vi "S2C_VLFT10_Proc_WaitForReboot.vi"(7 "Timeout":dbl, 8 "Error In":errorcluster, 11 "State":string) -> (0 "Error Out":errorcluster, 3 "Result":string)   [LabVIEW 2015]
uses:
  Fornax/VIs/PolyDriver/Typedefs/ExternalCommClient.ctl
  Fornax/VIs/PolyDriver/Typedefs/SystemState.ctl
  Fornax/VIs/S2C_FORNAX_Proc_Globals.vi
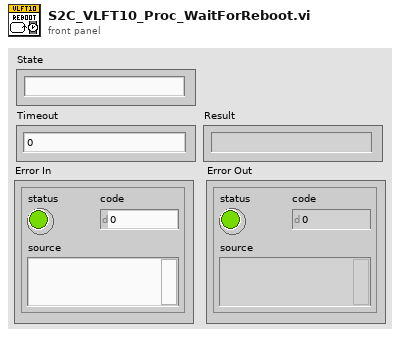
[diagram p1: front panel]
types:
  T1 = typedef "ExternalCommClient.ctl" = i16
  T2 = cluster{"ClientType":T1, "PostDelay (ms)":i32, "ClearFornaxMsgs":bool}
  T3 = cluster{"Partition":string, "Message":string, "M_ClientType":T1, "M_ClientId":string, "M_ResponseVersion":string, "M_ControllerBoardId":string, "M_ResponseValue":string, "M_ClientAlias":string, "M_ResponseOptions":string, "M_ClientIpAddress":string, "M_Crc32":i32}
  T4 = cluster{"Partition":string, "Message":string, "M_ClientType":T1, "M_ClientId":string, "M_ResponseVersion":string, "M_ControllerBoardId":string, "M_ResponseValue":string, "M_ClientAlias":string, "M_ResponseOptions":string, "M_ClientIpAddress":string}
  T5 = typedef "SystemState.ctl" = i16
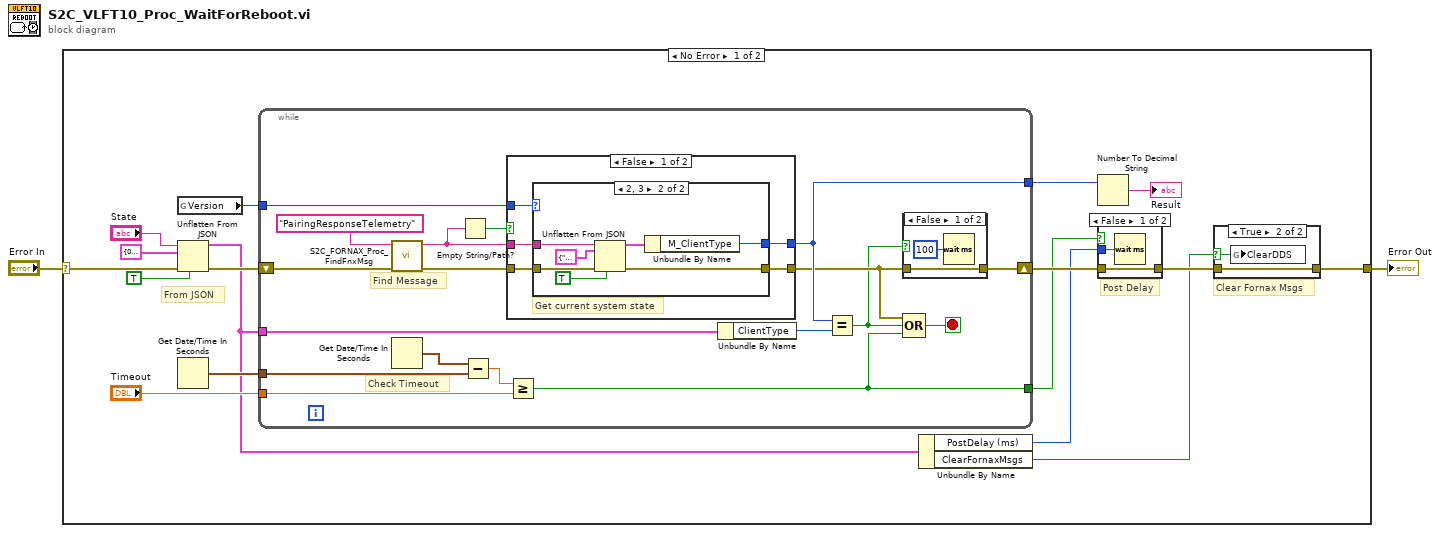
[diagram p0: block diagram]
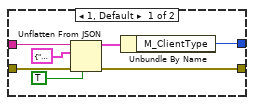
[diagram p5: hidden frame]
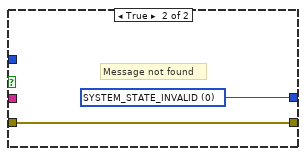
[diagram p6: hidden frame]
diagram:
  n1 = case shown="No Error" "Error In" {
    selector: "Error In" -> [w16 w68]
    tunnel: [w5 w68] -> w1
    frame No Error {
      # "Clear Fornax Msgs"
      # "Post Delay"
      # "From JSON"
      n2 = global read "S2C_FORNAX_Proc_Globals.vi" "Version"() -> (w19:i32)
      n3 = Unflatten From JSON(JSON string="State", type and defaults=T2 {"ClientType"=0, "PostDelay (ms)"=0, "ClearFornaxMsgs"=FALSE}, default null elements? (F)=TRUE, error in (no error)=w16) -> (value=w10:T2, error out=w15:errorcluster)  [unwired: 3 in]
      n4 = Get Date/Time In Seconds() -> (seconds since 1Jan1904=w14:timestamp)
      n5 = while {
        tunnel: w19 -> [w42]
        tunnel: w10 -> [w40]
        shift-right: [w29] -> w9
        shift-left: w15 -> [w41]
        tunnel: w14 -> [w36]
        tunnel: "Timeout" -> [w35]
        tunnel: [w31] -> w12
        tunnel: [w27] -> w8
        stop <- w32 stop-if-true
        # "Check Timeout"
        # "Find Message"
        n6 = call "S2C_FORNAX_Proc_FindFnxMsg.vi"("Error In"=w41, "MsgName"="PairingResponseTelemetry") -> ("Error Out"=w43:errorcluster, "Message"=w38:string)  [unwired: 8 in]
        n7 = Get Date/Time In Seconds() -> (seconds since 1Jan1904=w37:timestamp)
        n8 = Empty String/Path?(string/path=w38) -> (empty?=w39:bool)
        n9 = Subtract(x=w37, y=w36) -> (x-y=w34:dbl)
        n10 = case shown="False" w39 {
          tunnel: w43 -> [w51 w67]
          tunnel: w42 -> [w50 _]
          tunnel: [w49 w67] -> w30
          tunnel: [w48 w66] -> w31
          tunnel: w38 -> [w47 _]
          frame False {
            # "Get current system state"
            n11 = case shown="2, 3" w50 {
              tunnel: w51 -> [w57 w64]
              tunnel: [w55 w62] -> w49
              tunnel: [w54 w61] -> w48
              tunnel: w47 -> [w53 w60]
              frame 1, Default {
                n12 = Unflatten From JSON(JSON string=w53, type and defaults=T3 {"Partition"="", "Message"="", "M_ClientType"=0, "M_ClientId"="", "M_ResponseVersion"="", "M_ControllerBoardId"="", "M_ResponseValue"="", "M_ClientAlias"="", "M_ResponseOptions"="", "M_ClientIpAddress"="", "M_Crc32"=0}, default null elements? (F)=TRUE, error in (no error)=w57) -> (value=w56:T3, error out=w55:errorcluster)  [unwired: 3 in]
                n13 = Unbundle By Name(w56) -> ("M_ClientType"=w54:T1)
              }
              frame 2, 3 {
                n14 = Unflatten From JSON(JSON string=w60, type and defaults=T4 {"Partition"="", "Message"="", "M_ClientType"=0, "M_ClientId"="", "M_ResponseVersion"="", "M_ControllerBoardId"="", "M_ResponseValue"="", "M_ClientAlias"="", "M_ResponseOptions"="", "M_ClientIpAddress"=""}, default null elements? (F)=TRUE, error in (no error)=w64) -> (value=w63:T4, error out=w62:errorcluster)  [unwired: 3 in]
                n15 = Unbundle By Name(w63) -> ("M_ClientType"=w61:T1)
              }
            }
          }
          frame True {
            w66 = T5 0 items=["SYSTEM_STATE_INVALID", "SYSTEM_STATE_INIT", "SYSTEM_STATE_POST", "SYSTEM_STATE_CLINICAL", "SYSTEM_STATE_SERVICE", "SYSTEM_STATE_SW_UPDATE", "SYSTEM_STATE_SHUTDOWN", "SYSTEM_STATE_CALIBRATION", "SYSTEM_STATE_CONFIGURATION", "SYSTEM_STATE_CLINICAL_CONFIGURATION"] ("M_SystemState")
            # "Message not found"
          }
        }
        n16 = Greater Or Equal?(x=w34, y=w35) -> (x >= y?=w27:bool)
        n17 = Unbundle By Name(w40) -> ("ClientType"=w33:T1)
        n18 = Equal?(x=w31, y=w33) -> (x = y?=w28:bool)
        n19 = case shown="False" w28 {
          tunnel: w30 -> [w45 w46]
          tunnel: [w45 w46] -> w29
          frame False {
            n20 = Wait (ms)(milliseconds to wait=u32 100) -> ()  [unwired: 1 out]
          }
          frame True {
          }
        }
        n21 = Compound Arithmetic op=OR(w30, w28, w27) -> (w32:bool)
      }
      n22 = Unbundle By Name(w10) -> ("PostDelay (ms)"=w7:i32, "ClearFornaxMsgs"=w4:bool)
      n23 = Number To Decimal String(number=w12) -> (decimal integer string=→"Result":string)  [unwired: 1 in]
      n24 = case shown="False" w8 {
        tunnel: w9 -> [w24 w25]
        tunnel: [w24 w25] -> w6
        tunnel: w7 -> [w23 _]
        frame False {
          n25 = Wait (ms)(milliseconds to wait=w23) -> ()  [unwired: 1 out]
        }
        frame True {
        }
      }
      n26 = case shown="True" w4 {
        selector: w4 -> [_ w21]
        tunnel: w6 -> [w20 w22]
        tunnel: [w20 w22] -> w5
        frame False {
        }
        frame True {
          n27 = global write "S2C_FORNAX_Proc_Globals.vi" "ClearDDS"(w21) -> ()
        }
      }
    }
    frame Error {
    }
  }
  "Error Out" <- w1
